vi "Prober_ProbeTouchdown.vi"(8 "error in (no error)":errorcluster, 11 "TeslaVeloxProbeStation in":refnum<class "TeslaVeloxProbeStation.lvclass">) -> (0 "error out":errorcluster, 1 "previous Z [µm]":i32, 2 "Z [µm]":i32, 3 "TeslaVeloxProbeStation out":refnum<class "TeslaVeloxProbeStation.lvclass">)   [LabVIEW 2018, in "TeslaVeloxProbeStation.lvclass"]
uses:
  TeslaVeloxProbeStation.lvclass
  TeslaVeloxProbeStation.lvclass/TeslaVeloxProbeStation.ctl
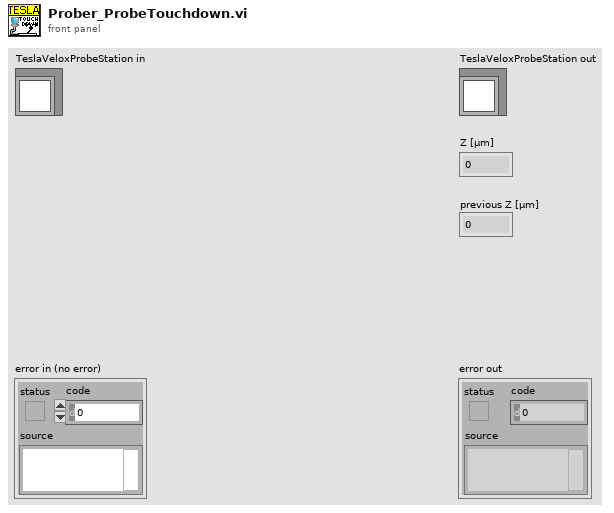
[diagram p1: front panel]
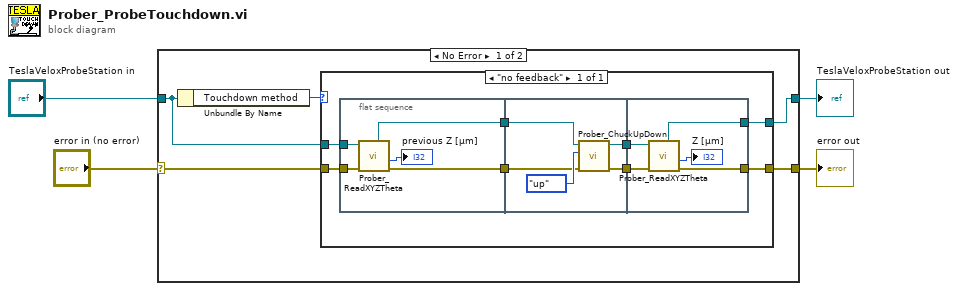
[diagram p0: block diagram]
diagram:
  n1 = case shown="No Error" "error in (no error)" {
    selector: "error in (no error)" -> [w7 w34]
    tunnel: "TeslaVeloxProbeStation in" -> [w8 w33]
    tunnel: [w6 w33] -> w2
    tunnel: [w5 w34] -> w1
    frame No Error {
      n2 = Unbundle By Name(w8) -> ("Touchdown method"=w9:enum16{"no feedback"})
      n3 = case shown="\"no feedback\"" w9 {
        tunnel: w8 -> [w17]
        tunnel: w7 -> [w16]
        tunnel: [w11] -> w6
        tunnel: [w10] -> w5
        frame "no feedback" {
          n4 = flat-sequence {
            tunnel: w17 -> [w20]
            tunnel: w16 -> [w22]
            tunnel: [w19] -> w15
            tunnel: [w18] -> w14
            tunnel: w15 -> [w26]
            tunnel: w14 -> [w25]
            tunnel: [w24] -> w13
            tunnel: [w23] -> w12
            tunnel: w13 -> [w32]
            tunnel: w12 -> [w31]
            tunnel: [w29] -> w11
            tunnel: [w28] -> w10
            frame #0 {
              n5 = call-dynamic "Prober_ReadXYZTheta.vi"("error in (no error)"=w22, "TeslaVeloxProbeStation in"=w20) -> ("error out"=w19:errorcluster, "Z location [µm]"=→"previous Z [µm]":i32, "TeslaVeloxProbeStation out"=w18:refnum<class "TeslaVeloxProbeStation.lvclass">)  [unwired: 4 in, 3 out]
            }
            frame #1 {
              n6 = call-dynamic "Prober_ChuckUpDown.vi"("error in (no error)"=w26, "Direction"=enum16{"up", "down"}."up", "TeslaVeloxProbeStation in"=w25) -> ("error out"=w23:errorcluster, "TeslaVeloxProbeStation out"=w24:refnum<class "TeslaVeloxProbeStation.lvclass">)  [unwired: 6 in, 1 out]
            }
            frame #2 {
              n7 = call-dynamic "Prober_ReadXYZTheta.vi"("error in (no error)"=w31, "TeslaVeloxProbeStation in"=w32) -> ("error out"=w28:errorcluster, "Z location [µm]"=→"Z [µm]":i32, "TeslaVeloxProbeStation out"=w29:refnum<class "TeslaVeloxProbeStation.lvclass">)  [unwired: 4 in, 3 out]
            }
          }
        }
      }
    }
    frame Error {
    }
  }
  "error out" <- w1
  "TeslaVeloxProbeStation out" <- w2
